vi "Test_bool_conversion.vi"() -> ()   [LabVIEW 2018]
panel:
  in  "4":bool=TRUE
  out "Value":u32
  in  "3":bool=TRUE
  in  "2":bool=TRUE
  in  "1":bool=TRUE
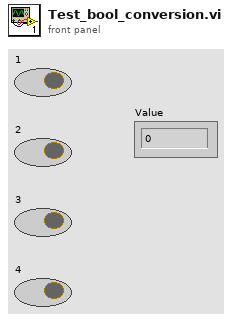
[diagram p1: front panel]
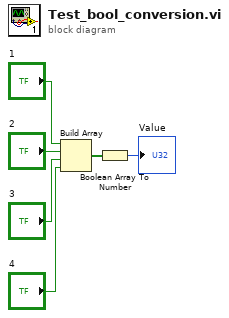
[diagram p0: block diagram]
diagram:
  n1 = Build Array("1", "2", "3", "4") -> (w6:bool[])
  n2 = Boolean Array To Number(Boolean array=w6) -> (number=→"Value":u32)
